vi "decodeStream.vi"(8 "error in (no error)":errorcluster, 9 "beginIndex":i32, 10 "binary stream":u8[](array[numeric]), 11 "tBSONArray in":refnum<class "tBSONArray.lvclass">) -> (0 "error out":errorcluster, 1 "endIndex":i32, 2 "binary stream out":u8[](array[numeric]), 3 "tBSONArray out":refnum<class "tBSONArray.lvclass">)   [LabVIEW 2013, in "BSON.lvlib" / "tBSONArray.lvclass"]
uses:
  tBSONArray.lvclass
  tBSONElement/tBSONElement.lvclass
  tBSONDocument/getElements.vi
  setValue.vi
  tBSONDocument/tBSONDocument.lvclass
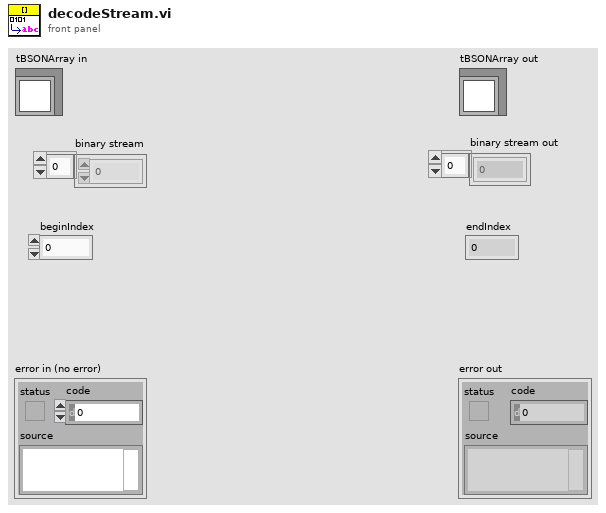
[diagram p1: front panel]
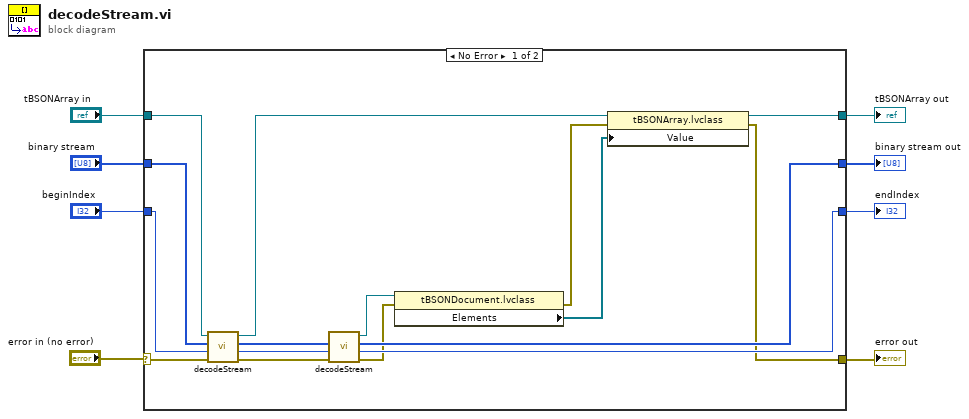
[diagram p0: block diagram]
diagram:
  n1 = case shown="No Error" "error in (no error)" {
    selector: "error in (no error)" -> [w24 w27]
    tunnel: [w10 w27] -> w7
    tunnel: "tBSONArray in" -> [w23 w28]
    tunnel: "binary stream" -> [w22 w25]
    tunnel: "beginIndex" -> [w21 w26]
    tunnel: [w9 w28] -> w3
    tunnel: [w16 w26] -> w2
    tunnel: [w17 w25] -> w1
    frame No Error {
      n2 = call-parent "decodeStream.vi"("error in (no error)"=w24, "beginIndex"=w21, "binary stream"=w22, "tBSONElement in"=w23) -> ("error out"=w20:errorcluster, "endIndex"=w18:i32, "binary stream out"=w19:u8[], "tBSONElement out"=w15:refnum<class "tBSONArray.lvclass">)  [unwired: 4 in]
      n3 = call "decodeStream.vi"("error in (no error)"=w20, "Begin Index"=w18, "Byte Data In"=w19) -> ("error out"=w13:errorcluster, "End Index"=w16:i32, "Byte Data Out"=w17:u8[], "tBSONDocument out"=w14:refnum<class "tBSONDocument.lvclass">)  [unwired: 5 in]
      n4 = property class="tBSONDocument.lvclass"(reference=w14, error in=w13) -> (error out=w11:errorcluster, "Elements"=w12:refnum<class "tBSONElement.lvclass">[])  [unwired: 1 out]
      n5 = property class="tBSONArray.lvclass"(reference=w15, error in=w11, "Value"=w12) -> (reference out=w9:refnum<class "tBSONArray.lvclass">, error out=w10:errorcluster)
    }
    frame Error {
    }
  }
  "error out" <- w7
  "tBSONArray out" <- w3
  "binary stream out" <- w1
  "endIndex" <- w2
